vi "Wait for Trigger State_Next State Decision.vi"(7 "End of Acquisition":bool=TRUE, 10 "Acq Hold=0?":bool=TRUE, 11 "Reference Trigger":bool=TRUE) -> (3 "Next State":T1=enum."Wait for Trigger")   [LabVIEW 2014]
uses:
  Acquisition Engine State.ctl
panel:
  # "Copyright 2014 Vidrio Technologies\nScanImage 5 software is licensed under the Apache License, Version 2.0 (the \"License\"); you may not use any files contained\nwithin the ScanImage 5 release except in compliance with the License. You may obtain a copy of the License at\n http://www.apache.org/licenses/LICENSE-2.0\nUnless required by applicable law or agreed to in writing, software distributed under the License is distributed on an\n\"AS IS\" BASIS, WITHOUT WARRANTIES OR CONDITIONS OF ANY KIND, either express or implied. See the License for the\n specific language governing permissions and limitations under the License."
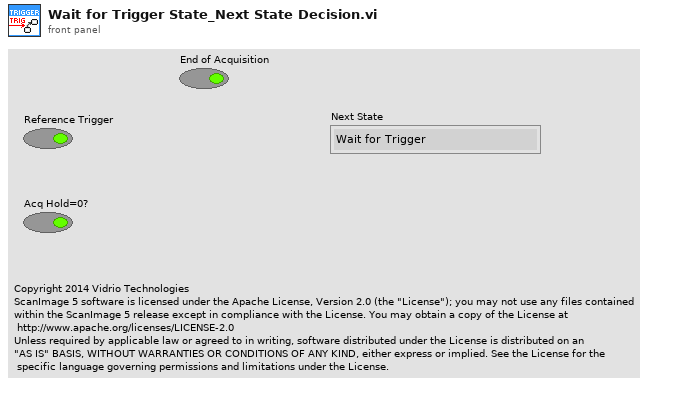
[diagram p1: front panel]
types:
  T1 = typedef "Acquisition Engine State.ctl" = enum8{"Idle", "Wait for Trigger", "Acquisition Hold Off Time", "Read Data", "Check Frame Done", "Check Grab Done", "Check Acquisition Done", "Wait Flyback Periods", "Flush Data"}
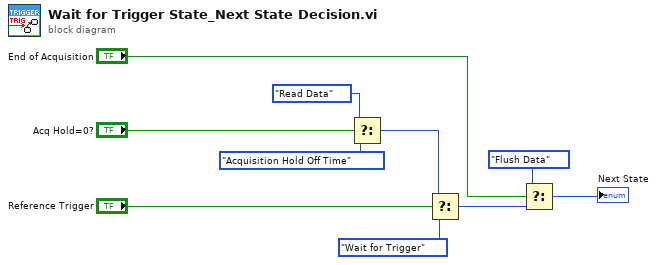
[diagram p0: block diagram]
diagram:
  n1 = Select(t=Acquisition_Engine_State."Read Data" ("Acquisition Engine State"), s="Acq Hold=0?", f=Acquisition_Engine_State."Acquisition Hold Off Time") -> (s? t:f=w7:T1)
  n2 = Select(t=w7, s="Reference Trigger", f=Acquisition_Engine_State."Wait for Trigger") -> (s? t:f=w4:T1)
  n3 = Select(t=Acquisition_Engine_State."Flush Data", s="End of Acquisition", f=w4) -> (s? t:f=→"Next State":T1)
